vi "Substitute Message.vi"(10 "Message to Substitute":refnum<class "MSG.lvclass">) -> (3 "Translator":refnum<class "SubstututeMessage.lvclass">)   [LabVIEW 2011, in "Messenging.lvlib" / "SubstututeMessage.lvclass"]
uses:
  SubstututeMessage.lvclass
  TextVarientMessage/MSG.lvclass
  SubstututeMessage.lvclass/SubstututeMessage.ctl
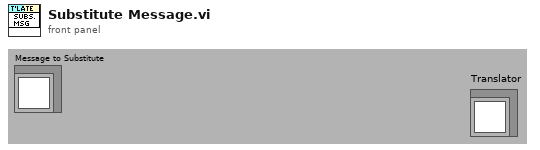
[diagram p1: front panel]
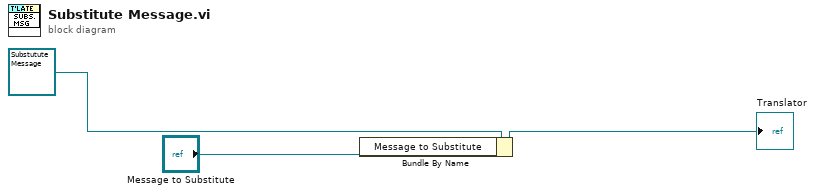
[diagram p0: block diagram]
diagram:
  n1 = Bundle By Name(cluster=refnum<class "SubstututeMessage.lvclass"> refnum ("SubstututeMessage in"), "Message to Substitute"="Message to Substitute") -> (→"Translator":refnum<class "SubstututeMessage.lvclass">)
